vi "Parse Library Items.vi"(0 "Library Path":path, 11 "error in (no error)":errorcluster) -> (4 "References":refnum<vi>[](array[refnum]), 6 "File Names":string[](array[string]), 8 "Display Name":string, 10 "Description":string, 15 "error out":errorcluster)   [LabVIEW 2016]
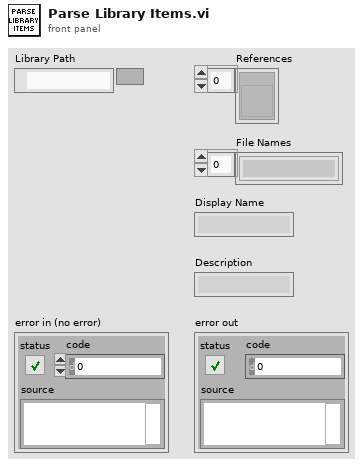
[diagram p1: front panel]
types:
  T1 = cluster{string, "filename without extension":string, "Reference":refnum<vi>}
  T2 = cluster{string, "filename without extension":string, "Reference":refnum<vi>}[]
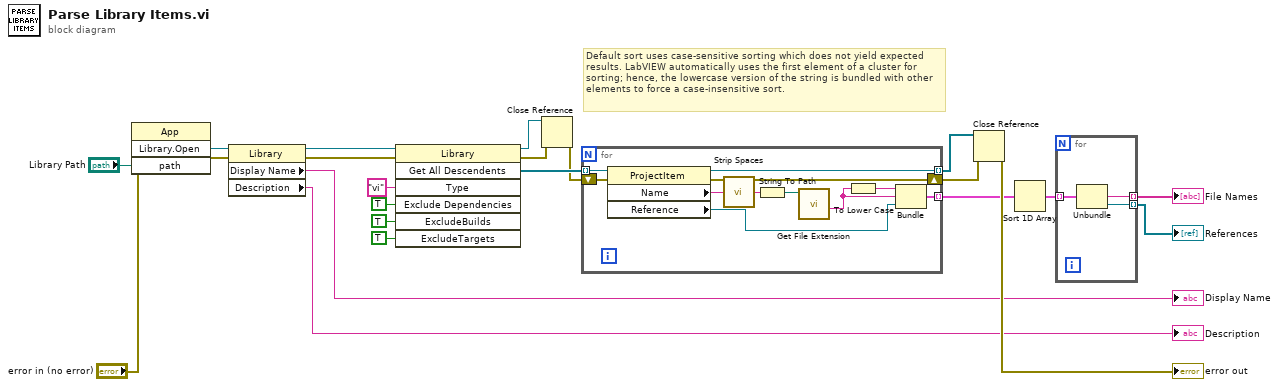
[diagram p0: block diagram]
diagram:
  # "Default sort uses case-sensitive sorting which does not yield expected results. LabVIEW automatically uses the first element of a cluster for sorting; hence, the lowercase version of the string is bundled with other elements to force a case-insensitive sort."
  n1 = invoke class="App" method="Library.Open"(error in="error in (no error)", "path"="Library Path") -> (error out=w8:errorcluster, "Open Library"=w13:refnum<vi>)  [unwired: 2 in, 2 out]
  n2 = property class="Library"(reference=w13, error in=w8) -> (reference out=w16:refnum<vi>, error out=w7:errorcluster, "Display Name"=→"Display Name":string, "Description"=→"Description":string)
  n3 = invoke class="Library" method="Get All Descendents"(reference=w16, error in=w7, "Type"="vi", "Exclude Dependencies"=TRUE ("ExcludeDependencies"), "ExcludeBuilds"=TRUE, "ExcludeTargets"=TRUE) -> (reference out=w22:refnum<vi>, error out=w10:errorcluster, "All Descendents"=w21:refnum<vi>[])  [unwired: 1 in, 4 out]
  n4 = Close Reference(reference=w22, error in (no error)=w10) -> (error out=w11:errorcluster)
  n5 = for {
    tunnel: w21 -> [w32] mode=indexing
    tunnel: [w31] -> w20 mode=indexing
    shift-right: [w33] -> w2
    shift-left: w11 -> [w34]
    tunnel: [w24] -> w3 mode=indexing
    n6 = property class="ProjectItem"(reference=w32, error in=w34) -> (reference out=w24:refnum<vi>, error out=w33:errorcluster, "Name"=w28:string, "Reference"=w25:refnum<vi>)
    n7 = call "Strip Spaces.vi"("String In"=w28) -> ("result string"=w30:string)  [unwired: 14 in]
    n8 = String To Path(string=w30) -> (path=w29:path)
    n9 = call <vilib>:"Get File Extension.vi"("file"=w29) -> ("filename without extension"=w27:string)  [unwired: 6 in, 4 out]
    n10 = To Lower Case(string=w27) -> (all lower case string=w26:string)
    n11 = Bundle(w26, "filename without extension"=w27, "Reference"=w25) -> (w31:T1)  [unwired: 1 in]
  }
  n12 = Close Reference(reference=w3, error in (no error)=w2) -> (error out=→"error out":errorcluster)
  n13 = Sort 1D Array(array=w20) -> (sorted array=w6:T2)
  n14 = for {
    tunnel: w6 -> [w37] mode=indexing
    tunnel: [w36] -> w5 mode=indexing
    tunnel: [w35] -> w4 mode=indexing
    n15 = Unbundle(w37) -> ("filename without extension"=w36:string, "Reference"=w35:refnum<vi>)  [unwired: 1 out]
  }
  "File Names" <- w5
  "References" <- w4
